vi "Read Message.vi"(8 "error in (no error)":errorcluster, 10 "Enable Header Information (False)":bool, 11 "VISA resource name":refnum<visa-resource-name>) -> (0 "error out":errorcluster, 2 "Message":string, 3 "VISA resource name out":refnum<visa-resource-name>)   [LabVIEW 2019, in "Stanford Research SIM900 Series.lvlib"]
doc: "Read message from the SIM900. If From Port is True the header information included when a message is sent from a port to the mainframe will be removed from the message."
uses:
  Stanford Research SIM900 Series.lvlib
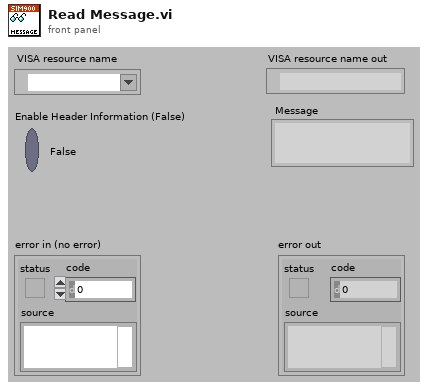
[diagram p1: front panel]
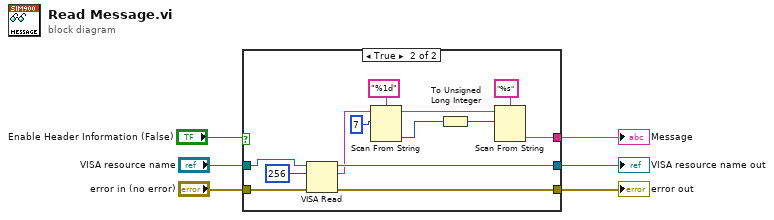
[diagram p0: block diagram]
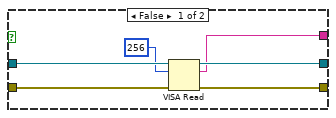
[diagram p2: hidden frame]
diagram:
  n1 = case shown="True" "Enable Header Information (False)" {
    tunnel: "VISA resource name" -> [w12 w25]
    tunnel: "error in (no error)" -> [w11 w24]
    tunnel: [w10 w23] -> w4
    tunnel: [w9 w22] -> w3
    tunnel: [w7 w14] -> w2
    frame False {
      n2 = VISA Read(VISA resource name=w12, byte count=u32 256, error in (no error)=w11) -> (VISA resource name out=w10:refnum<visa-resource-name>, read buffer=w7:string, error out=w9:errorcluster)  [unwired: 1 out]
    }
    frame True {
      n3 = VISA Read(VISA resource name=w25, byte count=u32 256, error in (no error)=w24) -> (VISA resource name out=w23:refnum<visa-resource-name>, read buffer=w20:string, error out=w22:errorcluster)  [unwired: 1 out]
      n4 = Scan From String(format string="%1d", input string=w20, initial scan location=u32 7) -> (remaining string=w15:string, output 1=w16:i32)  [unwired: 2 in, 2 out]
      n5 = To Unsigned Long Integer(number=w16) -> (unsigned 32bit integer=w13:u32)
      n6 = Scan From String(format string="%s", input string=w15, initial scan location=w13) -> (output 1=w14:string)  [unwired: 2 in, 3 out]
    }
  }
  "error out" <- w3
  "VISA resource name out" <- w4
  "Message" <- w2
